vi "Multi Instrument Do Core.vi"(8 "error in (no error)":errorcluster, 10 "Actor in":refnum<class "Actor.lvclass">, 11 "Instrument Msg in":refnum<class "Test Multi Instrument Msg.lvclass">) -> (0 "error out":errorcluster, 1 "Data":refnum<class "Data.lvclass">, 2 "Actor out":refnum<class "Actor.lvclass">, 3 "Instrument Msg out":refnum<class "Test Multi Instrument Msg.lvclass">)   [LabVIEW 2020, in "Test.lvlib" / "Test Multi Instrument Msg.lvclass"]
doc: "Message interaction with multiple instruments is handled by the Multi Instrument Do Core.\n\nMulti Instrument Msgs contains the Cores of all the Owners they require. Keep this in mind if the message wire is branched. Incorrect synchronization of nested Multi Instrument Msgs can lead to deadlocks if wire branching is used incorrectly!\n\nThe default implementation does nothing."
uses:
  Test Multi Instrument Msg.lvclass
  PPL/HDH.Actor Framework.Core.Actor.lvlibp/1abvi3w/vi.lib/ActorFramework/Actor/Actor.lvclass
  PPL/HDH.Data.Generic.lvlibp/Data.lvclass
  Test Instrument Msg/Test Instrument Msg.lvclass
  Data/Test Double Data/Test Double Data.lvclass
  C:/Current projects/WS/PPL/HDH.Data.Generic.lvlibp/Data.lvclass
  PPL/HDH.Data.Generic.lvlibp/Generic Data/Generic Data.lvclass
  PPL/HDH.Actor Framework.Core.Instrument Handler.lvlibp/Messages/Multi Instrument Msg/Multi Instrument Msg.lvclass
  C:/Current projects/WS/PPL/HDH.Actor Framework.Core.Instrument Handler.lvlibp/Messages/Instrument Msg/Instrument Msg.lvclass
  C:/Current projects/WS/PPL/HDH.Actor Framework.Core.Instrument Handler.lvlibp/Messages/Multi Instrument Msg/Multi Instrument Msg.lvclass
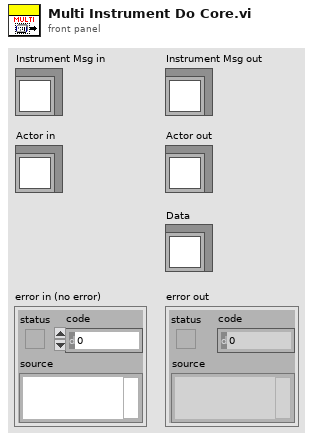
[diagram p1: front panel]
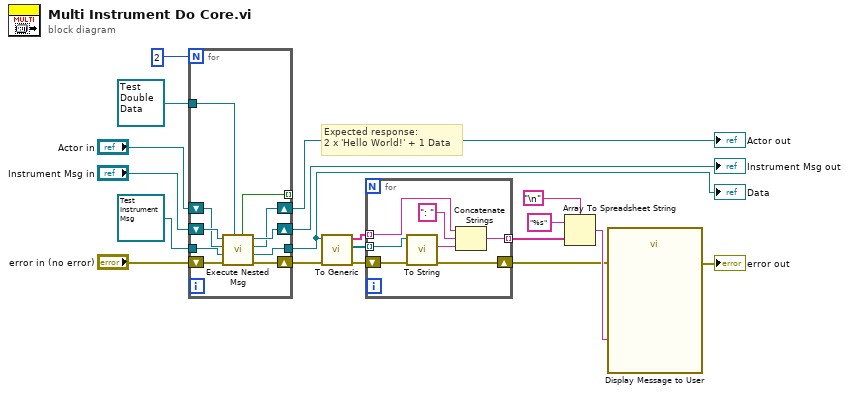
[diagram p0: block diagram]
diagram:
  # "Expected response:\n2 x 'Hello World!' + 1 Data"
  n1 = for {
    N: 2 -> [_]
    tunnel: refnum<class "Test Instrument Msg.lvclass"> refnum ("Test.lvlib:Test Instrument Msg.lvclass") -> [w28]
    tunnel: [w23] -> w11
    shift-right: [w22] -> w4
    shift-left: "error in (no error)" -> [w29]
    shift-right: [w26] -> w16
    shift-left: "Instrument Msg in" -> [w27]
    shift-right: [w24] -> w14
    shift-left: "Actor in" -> [w25]
    tunnel: refnum<class "Test Double Data.lvclass"> refnum ("Test.lvlib:Test Double Data.lvclass") -> [w21]
    tunnel: [w20] -> _ mode=indexing
    n2 = call "Execute Nested Msg.vi"("Response Data Type"=w21, "error in (no error)"=w29, "Instrument Msg to Run"=w28, "Actor in"=w25, "Multi Instrument Msg in"=w27) -> ("error out"=w22:errorcluster, "Data"=w23:refnum<class "Test Double Data.lvclass">, "Actor out"=w24:refnum<class "Actor.lvclass">, "Multi Instrument Msg out"=w26:refnum<class "Test Multi Instrument Msg.lvclass">, "Success?"=w20:bool)  [unwired: 2 in]
  }
  "Instrument Msg out" <- w16
  "Actor out" <- w14
  "Data" <- w11
  n3 = call-dynamic "To Generic.vi"("error in (no error)"=w4, "Test Double Data in"=w11) -> ("error out"=w3:errorcluster, "Generic Data"=w9:refnum<class "Generic Data.lvclass">[], "Data Name"=w10:string[])  [unwired: 7 in]
  n4 = for {
    tunnel: w10 -> [w35] mode=indexing
    tunnel: w9 -> [w36] mode=indexing
    tunnel: [w32] -> w8 mode=indexing
    shift-right: [w30] -> w2
    shift-left: w3 -> [w31]
    n5 = call-dynamic "To String.vi"("error in (no error)"=w31, "Generic Data in"=w36) -> ("error out"=w30:errorcluster, "String"=w33:string)  [unwired: 8 in]
    n6 = Concatenate Strings(w35, ": " ("string"), w33) -> (w32:string)
  }
  n7 = Array To Spreadsheet String(delimiter (Tab)="\n", array=w8, 3:"%s" ("format string")) -> (spreadsheet string=w5:string)
  n8 = call "Display Message to User"("error in (no error)"=w2, "Message"=w5) -> ("error out"=→"error out":errorcluster)  [unwired: 8 in, 1 out]
